vi "LD File Export.vi"(3 "Input Cluster":T1, 5 "Save Data?":bool, 6 "Output Filename (stem)":path, 8 "Data Collection Mode":enum32{"Reference", "Sample"}(ring), 10 "Selected Reference Channel":enum32{"Channel 1", "Channel 2", "Channel 3"}(ring), 12 "Selected Sample Channel":enum32{"Channel 1", "Channel 2", "Channel 3"}(ring)) -> ()   [LabVIEW 2017, in "LD Reading.lvclass"]
uses:
  LD Reading.lvclass
  <vilib>/Utility/file.llb/Write Delimited Spreadsheet (DBL).vi
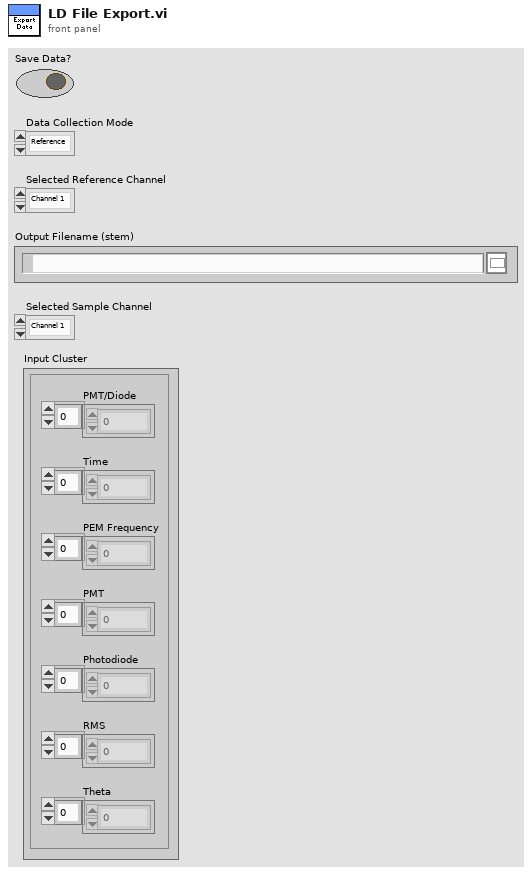
[diagram p1: front panel]
types:
  T1 = cluster{"Time":dbl[], "PMT":dbl[], "Photodiode":dbl[], "RMS":dbl[], "Theta":dbl[], "PEM Frequency":dbl[], "PMT/Diode":dbl[]}
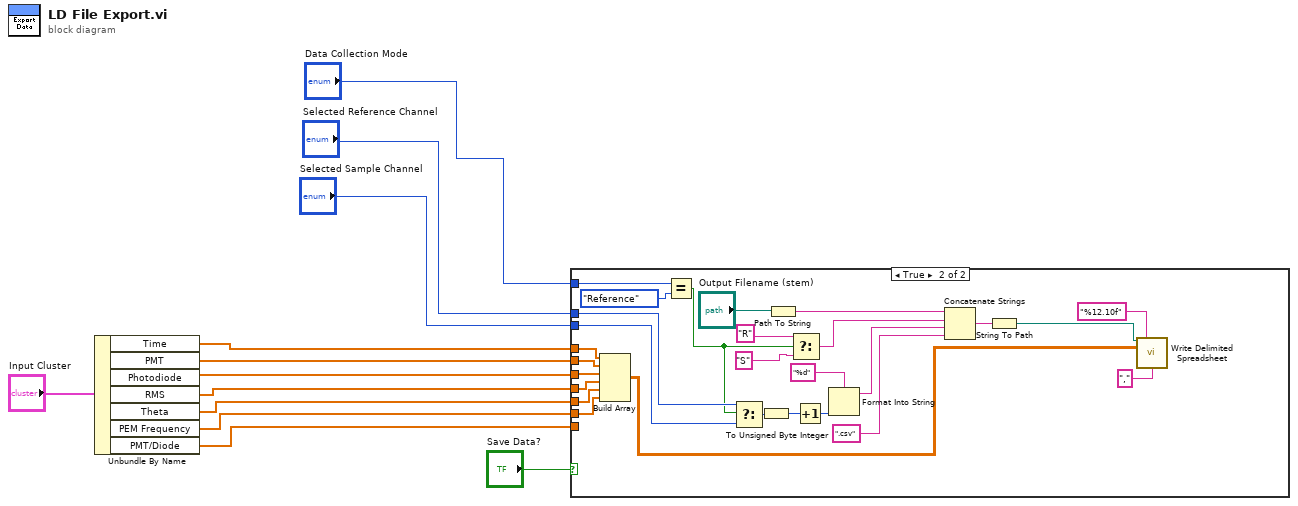
[diagram p0: block diagram]
diagram:
  n1 = Unbundle By Name("Input Cluster") -> ("Time"=w7:dbl[], "PMT"=w6:dbl[], "Photodiode"=w5:dbl[], "RMS"=w4:dbl[], "Theta"=w3:dbl[], "PEM Frequency"=w2:dbl[], "PMT/Diode"=w1:dbl[])
  n2 = case shown="True" "Save Data?" {
    tunnel: w6 -> [_ w18]
    tunnel: w7 -> [_ w19]
    tunnel: "Data Collection Mode" -> [_ w39]
    tunnel: "Selected Reference Channel" -> [_ w35]
    tunnel: "Selected Sample Channel" -> [_ w34]
    tunnel: w5 -> [_ w17]
    tunnel: w4 -> [_ w16]
    tunnel: w3 -> [_ w15]
    tunnel: w2 -> [_ w14]
    tunnel: w1 -> [_ _]
    frame False {
    }
    frame True {
      n3 = Build Array(w19, w18, w17, w16, w15, w14) -> (w25:dbl[][])
      n4 = Equal?(x=w39, y=enum32{"Reference", "Sample"}."Reference" ("Data Collection Mode")) -> (x = y?=w20:bool)
      n5 = Select(t=w35, s=w20, f=w34) -> (s? t:f=w31:enum32{"Channel 1", "Channel 2", "Channel 3"})
      n6 = To Unsigned Byte Integer(number=w31) -> (unsigned 8bit integer=w23:u8)
      n7 = Path To String(path="Output Filename (stem)") -> (string=w32:string)
      n8 = Select(t="R", s=w20, f="S") -> (s? t:f=w29:string)
      n9 = Increment(x=w23) -> (x+1=w22:u8)
      n10 = Format Into String(format string="%d", w22) -> (resulting string=w28:string)  [unwired: 2 in, 1 out]
      n11 = Concatenate Strings(w32, w29, w28, ".csv" ("string")) -> (w26:string)
      n12 = String To Path(string=w26) -> (path=w24:path)
      n13 = call-poly <vilib>:"Write Delimited Spreadsheet.vi"("file path (dialog if empty)"=w24, "format (%.3f)"="%12.10f", "2D data"=w25, "delimiter (\\t)"="," ("delimiter (\\t)")) -> ()  [unwired: 10 in, 2 out]
    }
  }
